vi "Update Next Coordinates.vi"(11 "Game Board in":refnum<class "Game Board.lvclass">) -> (3 "Game Board out":refnum<class "Game Board.lvclass">)   [LabVIEW 2024, in "Game Board.lvclass"]
doc: "MIT Licence\nCopyright (c) 2024 David Grollier"
uses:
  Game Board.lvclass
  Game Board.lvclass/Game Board.ctl
  Game Board Component/Movable/Movable.lvclass
  Game Componants.lvclass/Game Componants.ctl
  Game Board Component/Movable/Movable.lvclass/Movable.ctl
  Game Board Component/Game Board Component.lvclass
  Game Componants.lvclass
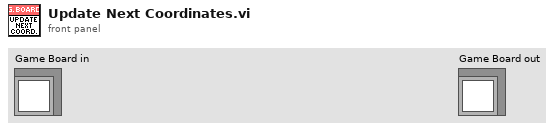
[diagram p1: front panel]
types:
  T1 = map{string, refnum<class "Game Board Component.lvclass">}
  T2 = typedef "Velocity.ctl" = cluster{"Vx":dbl, "Vy":dbl}
  T3 = typedef "Coordinates.ctl" = cluster{"x":dbl, "y":dbl}
  T4 = cluster{"Name":string, "Game Board Component":refnum<class "Game Board Component.lvclass">}
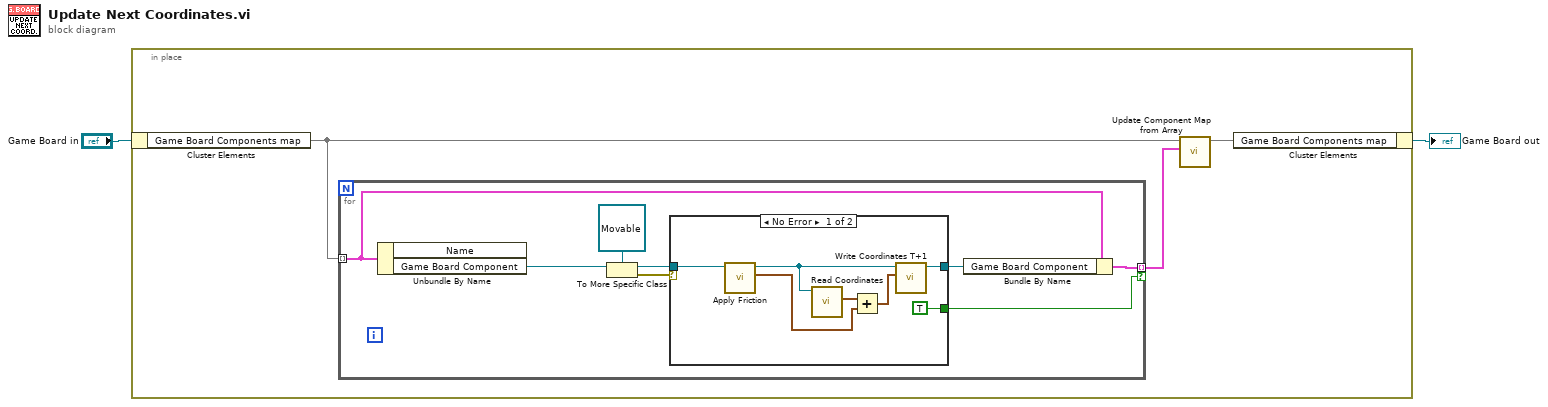
[diagram p0: block diagram]
diagram:
  n1 = in-place {
    n2 = in-place-cluster #1("Game Board in") -> ("Game Board Components map"=w5:T1)
    n3 = for {
      tunnel: w5 -> [w9] mode=indexing
      tunnel: [w7] -> w3 mode=indexing if=w6
      n4 = Unbundle By Name(w9) -> ("Game Board Component"=w10:refnum<class "Game Board Component.lvclass">)  [unwired: 1 out]
      n5 = To More Specific Class(target class=refnum<class "Movable.lvclass"> refnum ("Movable in"), reference=w10) -> (specific class reference=w13:refnum<class "Movable.lvclass">, error out=w11:errorcluster)  [unwired: 1 in]
      n6 = case shown="No Error" w11 {
        tunnel: w13 -> [w20 w21]
        tunnel: [w15 w21] -> w8
        tunnel: [TRUE _] -> w6
        frame No Error {
          n7 = call "Apply Friction.vi"("Movable in"=w20) -> ("Velocity out"=w18:T2, "Movable out"=w17:refnum<class "Movable.lvclass">)  [unwired: 9 in]
          n8 = call "Read Coordinates.vi"("Game Componants in"=w17) -> ("Coordinates"=w19:T3)  [unwired: 10 in]
          n9 = Add(x=w19, y=w18) -> (x+y=w16:T3)
          n10 = call "Write Coordinates T+1.vi"("Coordinates"=w16, "Movable in"=w17) -> ("Movable out"=w15:refnum<class "Movable.lvclass">)  [unwired: 9 in]
        }
        frame Error {
        }
      }
      n11 = Bundle By Name(cluster=w9, "Game Board Component"=w8) -> (w7:T4)
    }
    n12 = call "Update Component Map from Array.vi"("Array of components in"=w3, "Game Board Components[] in"=w5) -> ("Game Board Components[] out"=w4:T1)  [unwired: 9 in]
    n13 = in-place-cluster #1("Game Board Components map"=w4) -> (→"Game Board out":refnum<class "Game Board.lvclass">)
  }
